vi "End Receive Data.vi"(0 "Tovey9150 in":refnum<class "Tovey 9150.lvclass">, 11 "error in (no error)":errorcluster) -> (4 "Tovey9150 out":refnum<class "Tovey 9150.lvclass">, 6 "Data Present":bool, 8 "A":dbl, 10 "B":dbl, 15 "error out":errorcluster)   [LabVIEW 2015, in "Tovey 9150.lvclass"]
uses:
  Tovey 9150.lvclass
  Tovey 9150.lvclass/Tovey 9150.ctl
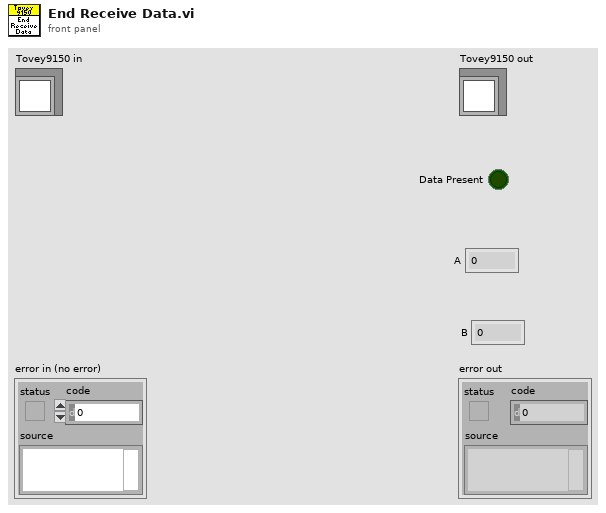
[diagram p1: front panel]
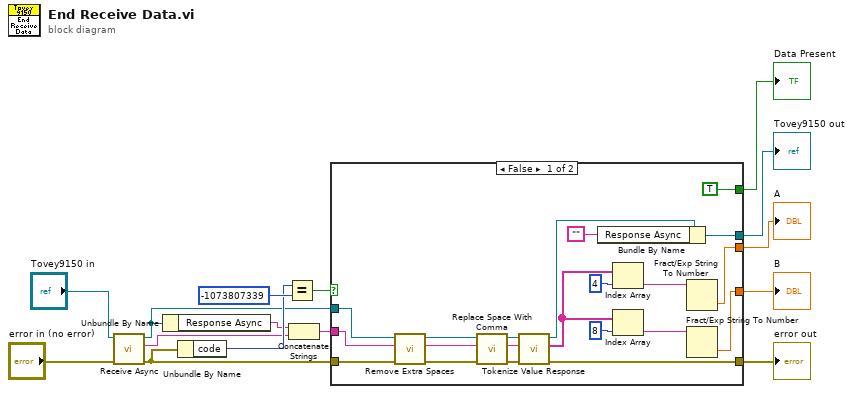
[diagram p0: block diagram]
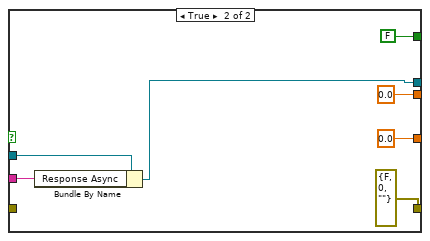
[diagram p2: hidden frame]
diagram:
  n1 = call "Receive Async.vi"("error in (no error)"="error in (no error)", "Tovey9150 in"="Tovey9150 in") -> ("error out"=w6:errorcluster, "Response"=w10:string, "Tovey9150 out"=w7:refnum<class "Tovey 9150.lvclass">)  [unwired: 7 in]
  n2 = Unbundle By Name(w7) -> ("Response Async"=w11:string)
  n3 = Unbundle By Name(w6) -> ("code"=w12:i32)
  n4 = Equal?(x=w12, y=-1073807339) -> (x = y?=w9:bool)
  n5 = Concatenate Strings(w11, w10) -> (w8:string)
  n6 = case shown="False" w9 {
    tunnel: w8 -> [w33 w39]
    tunnel: w7 -> [w36 w40]
    tunnel: w6 -> [w30 _]
    tunnel: [w27 errorcluster {"status"=FALSE, "code"=0, "source"=""} ("error out")] -> w2
    tunnel: [w21 0.0] -> w5
    tunnel: [w20 0.0] -> w4
    tunnel: [TRUE FALSE] -> w3
    tunnel: [w16 w38] -> w1
    frame False {
      n7 = call "Remove Extra Spaces.vi"("error in (no error)"=w30, "Input"=w33, "Tovey 9150 in"=w36) -> ("error out"=w29:errorcluster, "Output"=w32:string, "Tovey 9150 out"=w35:refnum<class "Tovey 9150.lvclass">)  [unwired: 6 in]
      n8 = call "Replace Space With Comma.vi"("error in (no error)"=w29, "Input"=w32, "Tovey 9150 in"=w35) -> ("error out"=w28:errorcluster, "Output"=w31:string, "Tovey 9150 out"=w34:refnum<class "Tovey 9150.lvclass">)  [unwired: 6 in]
      n9 = call "Tokenize Value Response.vi"("error in (no error)"=w28, "Input"=w31, "Tovey 9150 in"=w34) -> ("error out"=w27:errorcluster, "Tokens"=w24:string[], "Tovey 9150 out"=w18:refnum<class "Tovey 9150.lvclass">)  [unwired: 6 in]
      n10 = Bundle By Name(cluster=w18, "Response Async"="") -> (w16:refnum<class "Tovey 9150.lvclass">)
      n11 = Index Array(array=w24, index=4) -> (element=w22:string)
      n12 = Index Array(array=w24, index=8) -> (element=w23:string)
      n13 = Fract/Exp String To Number(string=w22) -> (number=w21:dbl)  [unwired: 3 in, 1 out]
      n14 = Fract/Exp String To Number(string=w23) -> (number=w20:dbl)  [unwired: 3 in, 1 out]
    }
    frame True {
      n15 = Bundle By Name(cluster=w40, "Response Async"=w39) -> (w38:refnum<class "Tovey 9150.lvclass">)
    }
  }
  "error out" <- w2
  "Tovey9150 out" <- w1
  "B" <- w4
  "A" <- w5
  "Data Present" <- w3
